vi "Pruebas-VER1.1.vi"() -> ()   [LabVIEW 2020]
uses:
  <vilib>/Instr/_visa.llb/VISA Open Access Mode.ctl
  <vilib>/Instr/_visa.llb/VISA Configure Serial Port (Instr).vi
panel:
  out "Numeric":i32
  in  "stop 2":bool
  in  "stop":bool
  out "Contador ciclos":i32
  in  "format string 3":string
  out "error out 2":errorcluster
  in  "Tab":enum32{"Datos Generales", "Calibración", "LVDT"}(tab) caption="Tab Control"
  in  "Número de muestra":string
  in  "Tab Control":enum32{"Contenido de Humedad ", " Anillo"}(tab)
  in  "Peso Tara (mr) [g]":string
  in  "Peso Suelo Seco + Tara (hora 1) (ms) [g]":string
  in  "Peso Suelo Seco + Tara (hora 0) (ms) [g]":string
  in  "Peso Suelo Húmedo + Tara (mh) [g]":string
  in  "Balanza N°":string
  in  "Cápsula N°":string
  in  "Balanza N°":string
  in  "Anillo N° [ANC-]":string
  in  "P. Anillo + muestra seca [g]":string
  in  "P. Anillo + Muestra sumergida [g]":string
  in  "P. Anillo + Muestra natural [g]":string
  in  "N° de brazo":string(combo)
  in  "Tipo de ensayo":string(combo)
  in  "Nombre del proyecto":string
  in  "Número de Ingreso":string
  in  "Operaria/o":string
  in  "Lugar donde se almacenará nuestro archivo":path
  in  "Save Button":bool
  in  "EST_CAL":string
  in  "Settings Button":bool
  in  "Nueva Configuración":dbl
  in  "Configuración":bool
  out "Hexadecimal":string
  out "Calibración Actual":dbl
  out "Defo (mm)":dbl
  out "microvolts":u32
  out "Voltaje (V)":dbl
  in  "Ingrese el valor de la carga":string
  in  "Obs Muestra":bool
  out "XY Graph":cluster{"X":dbl, "Y":dbl}[](graph)
  out "Actualización de tabla en tiempo real con deformación":string[][](table)
  in  "Observación de la muestra":string
  in  "Play Button":bool
  out "ciclo inicio":i32
  out "Voltaje (V) 2":dbl format="%#_8f"
  out "Deformación (mm)":dbl format="%#_6f"
  out "error out":errorcluster
  out "Microvolts":i32
  in  "Pause Button":bool
  in  "Cancel Button":bool
  # "Parámetros para calibración"
  # "Recuerde: Las observaciones van al final del ensayo para no perjudicar los demas datos"
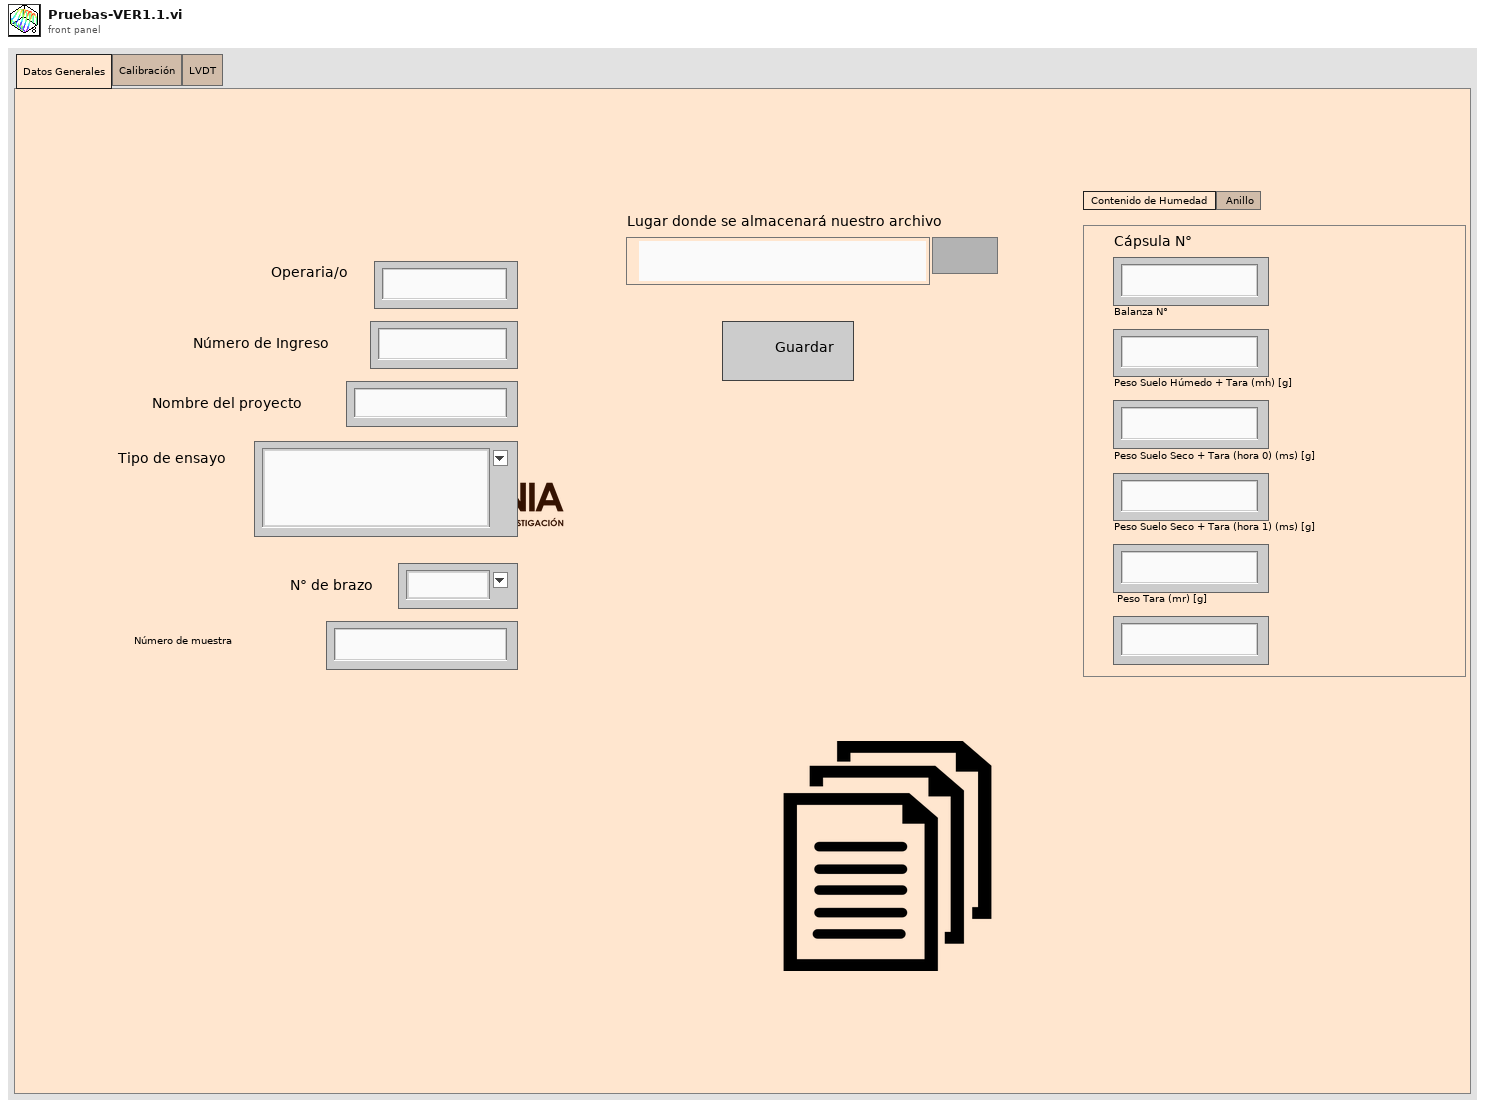
[diagram p1: front panel]
types:
  T1 = enum16{"open", "replace", "create", "open or create", "replace or create", "replace or create with confirmation"}
  T2 = typedef "VISA Open Access Mode.ctl" = u32
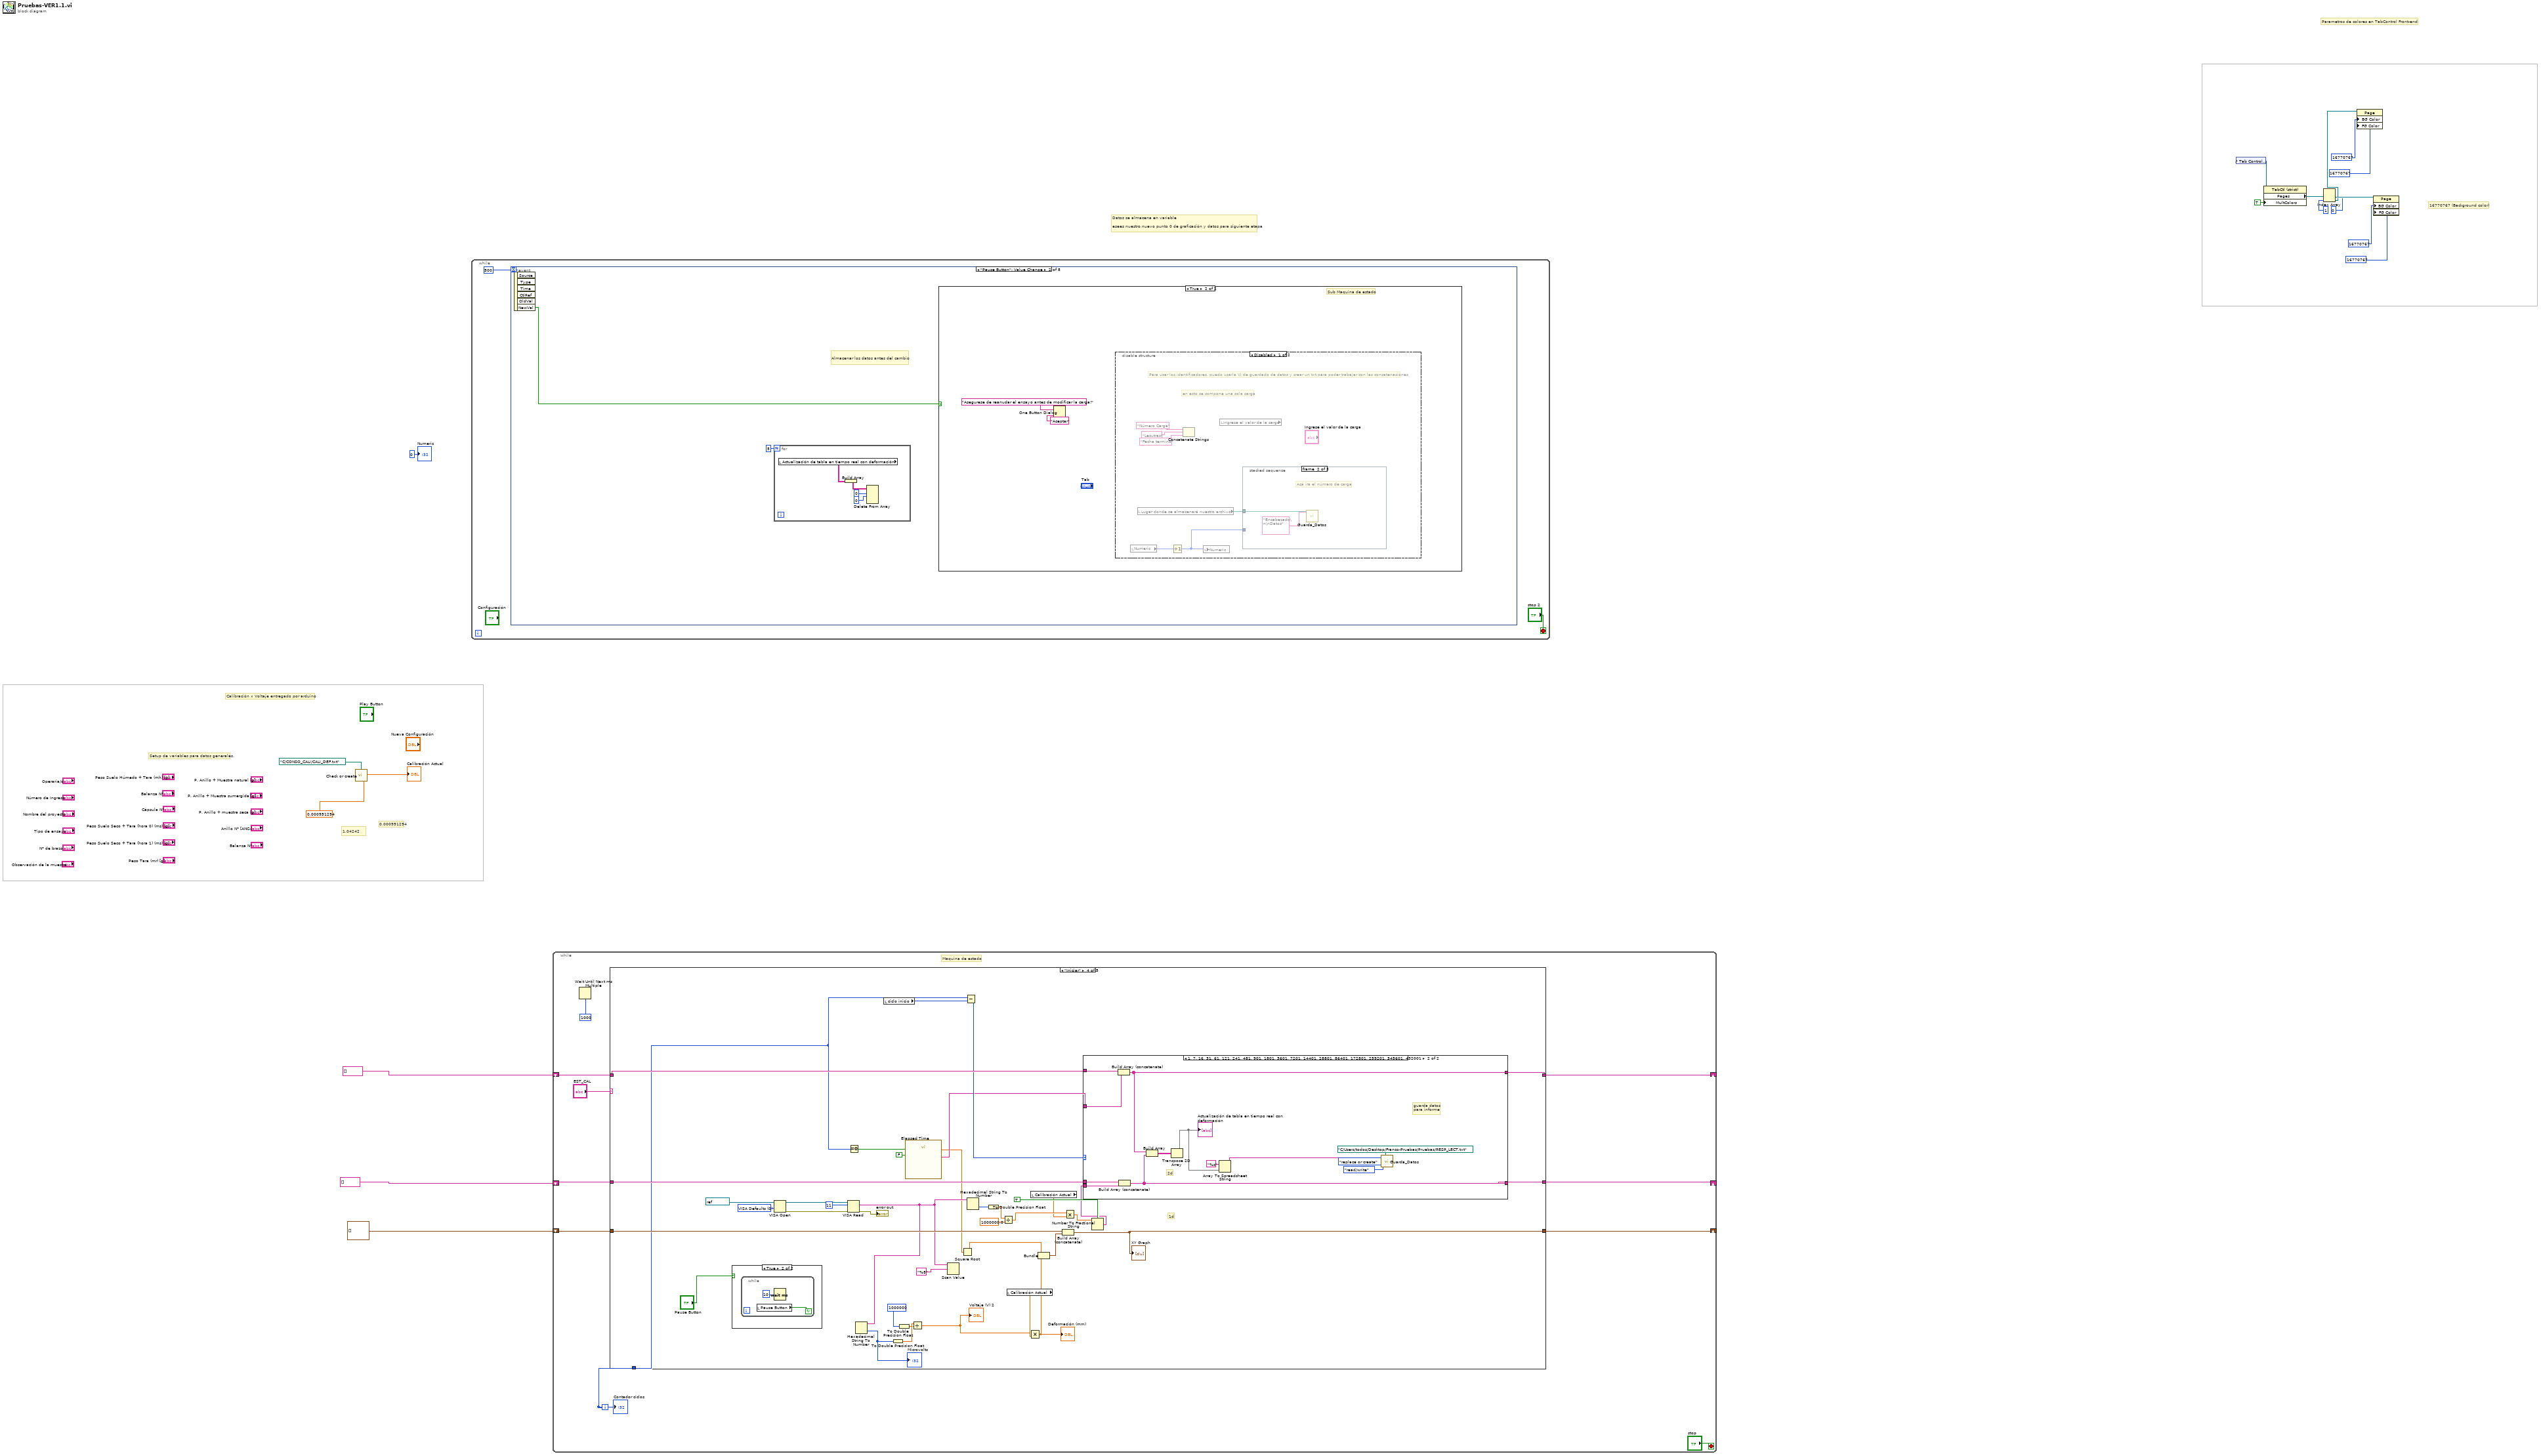
[diagram p0: block diagram]
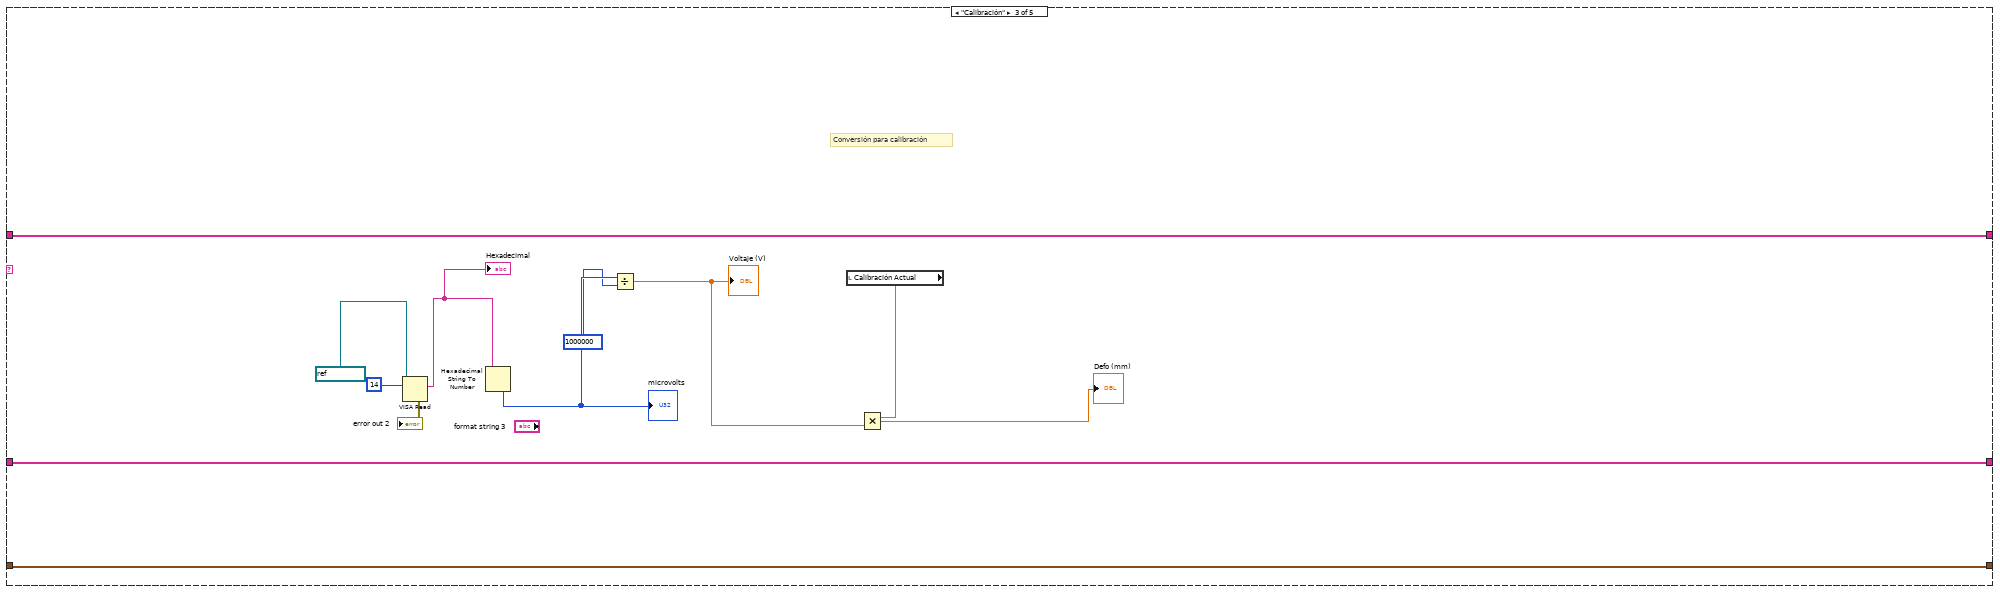
[diagram p4: hidden frame]
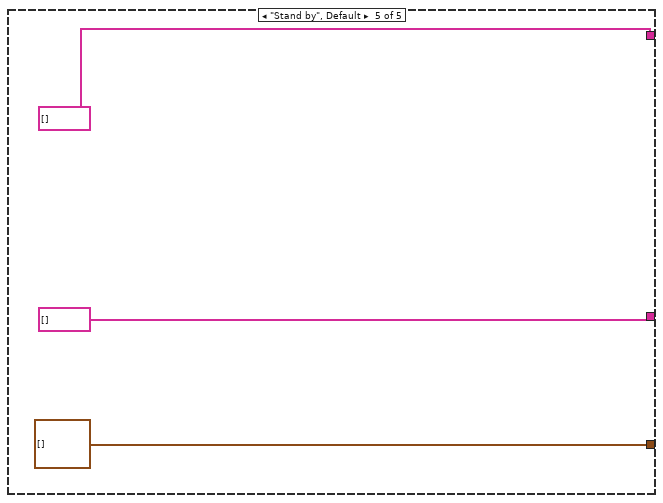
[diagram p7: hidden frame]
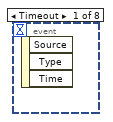
[diagram p8: hidden frame]
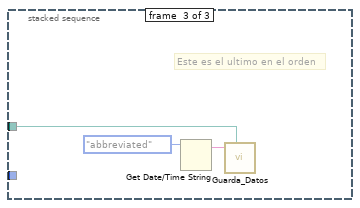
[diagram p11: hidden frame]
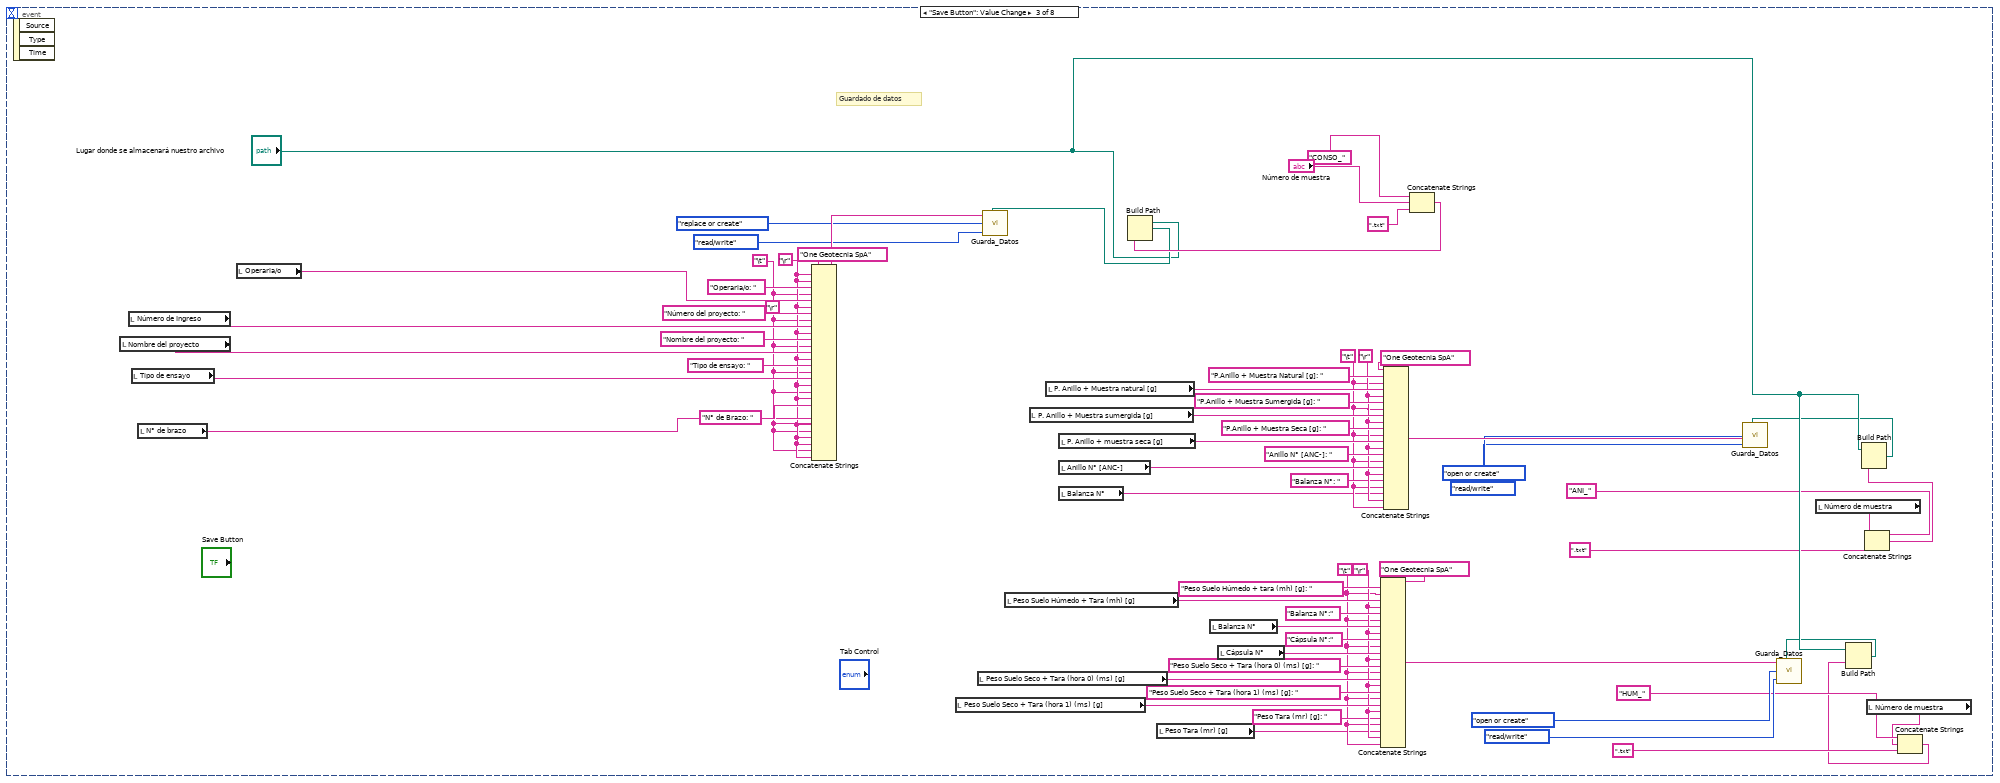
[diagram p13: hidden frame]
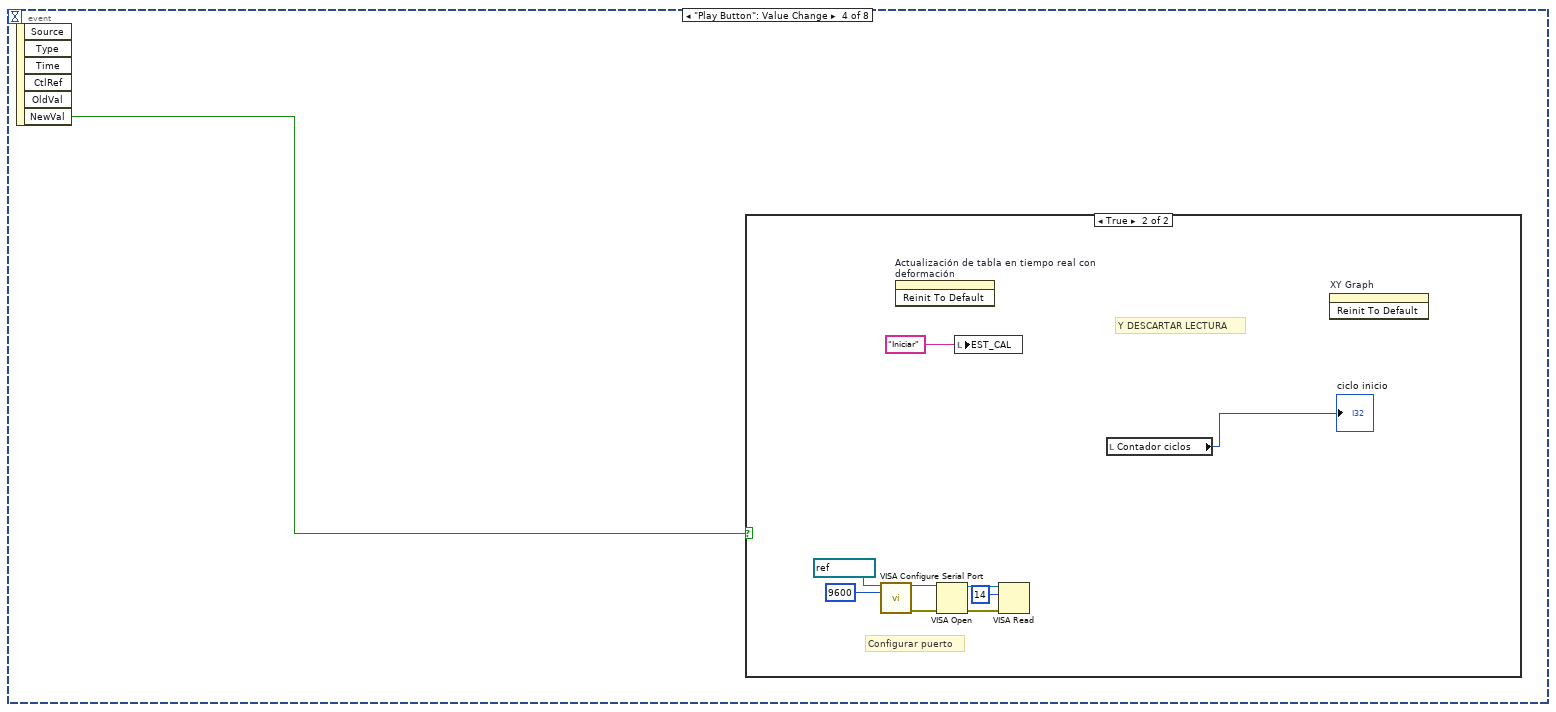
[diagram p14: hidden frame]
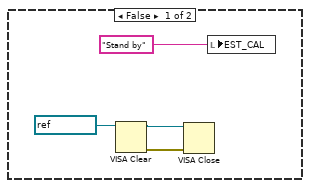
[diagram p15: hidden frame]
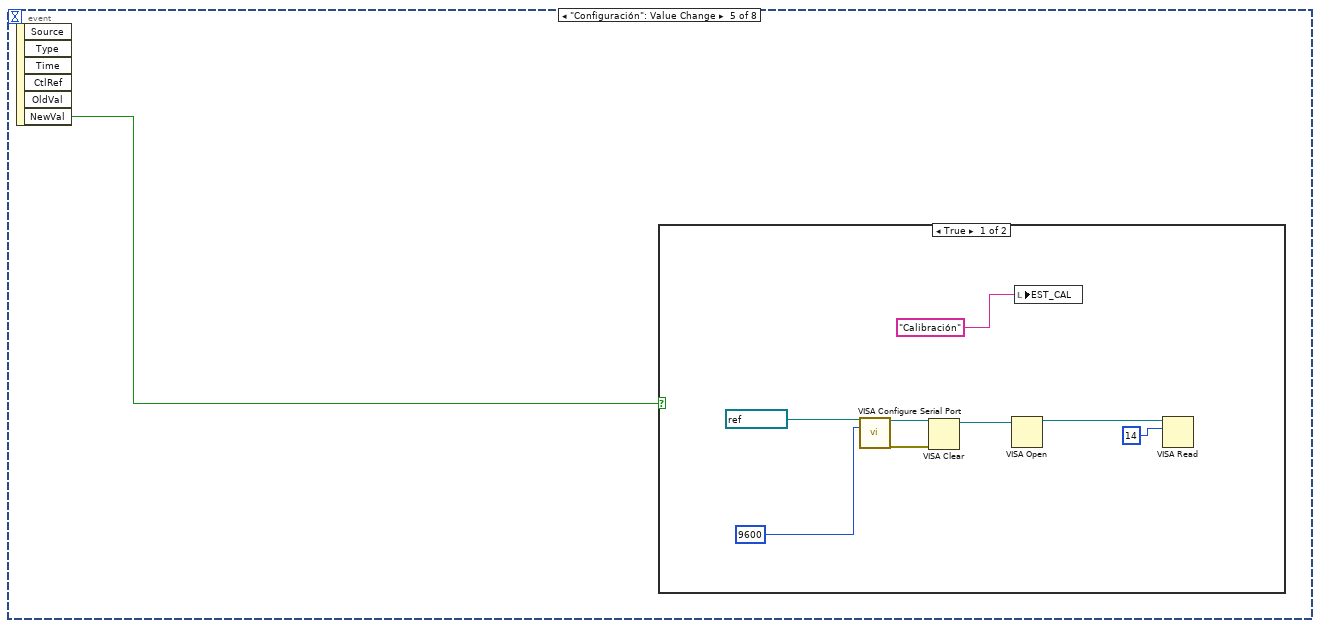
[diagram p16: hidden frame]
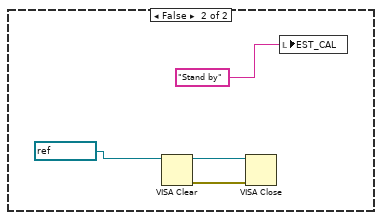
[diagram p17: hidden frame]
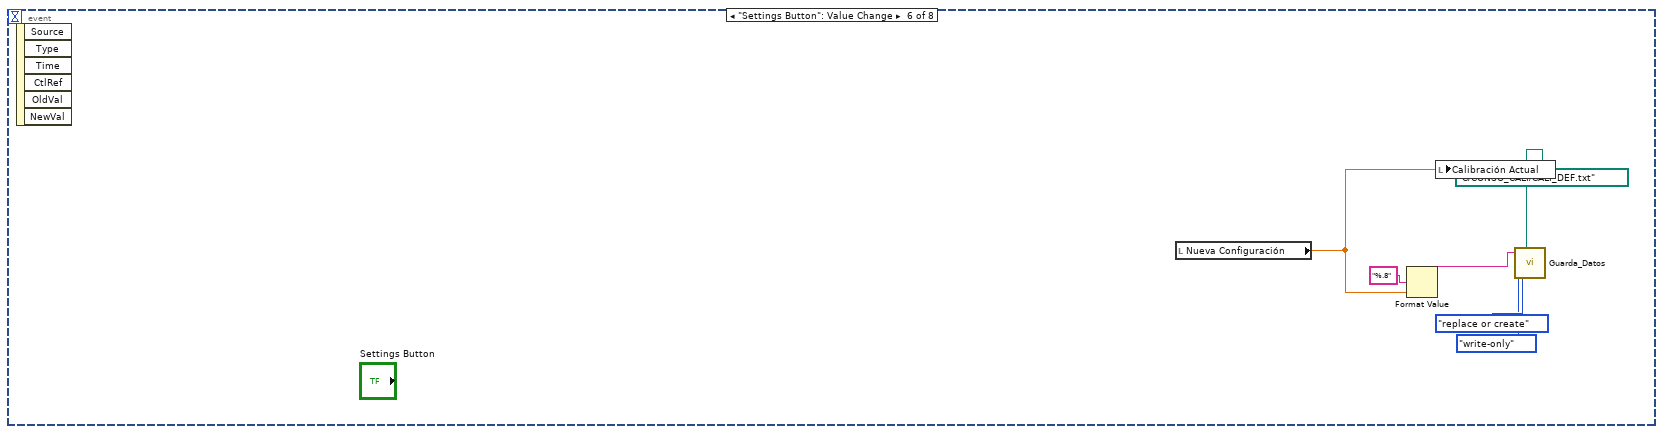
[diagram p18: hidden frame]
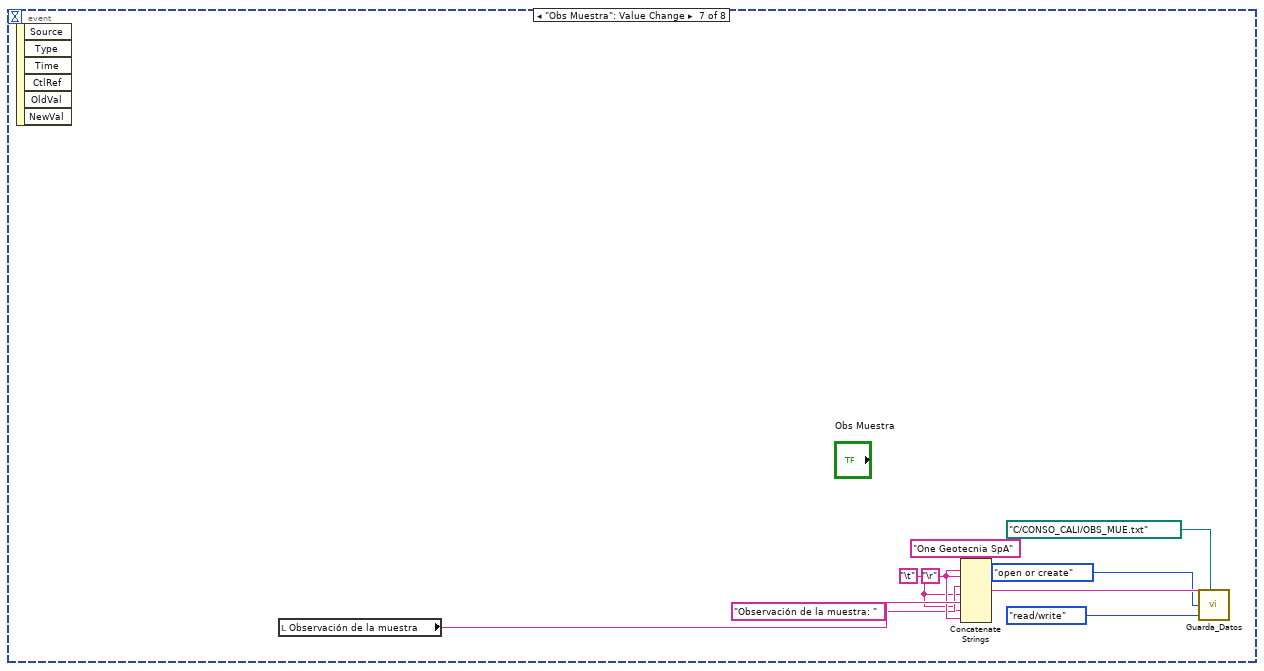
[diagram p19: hidden frame]
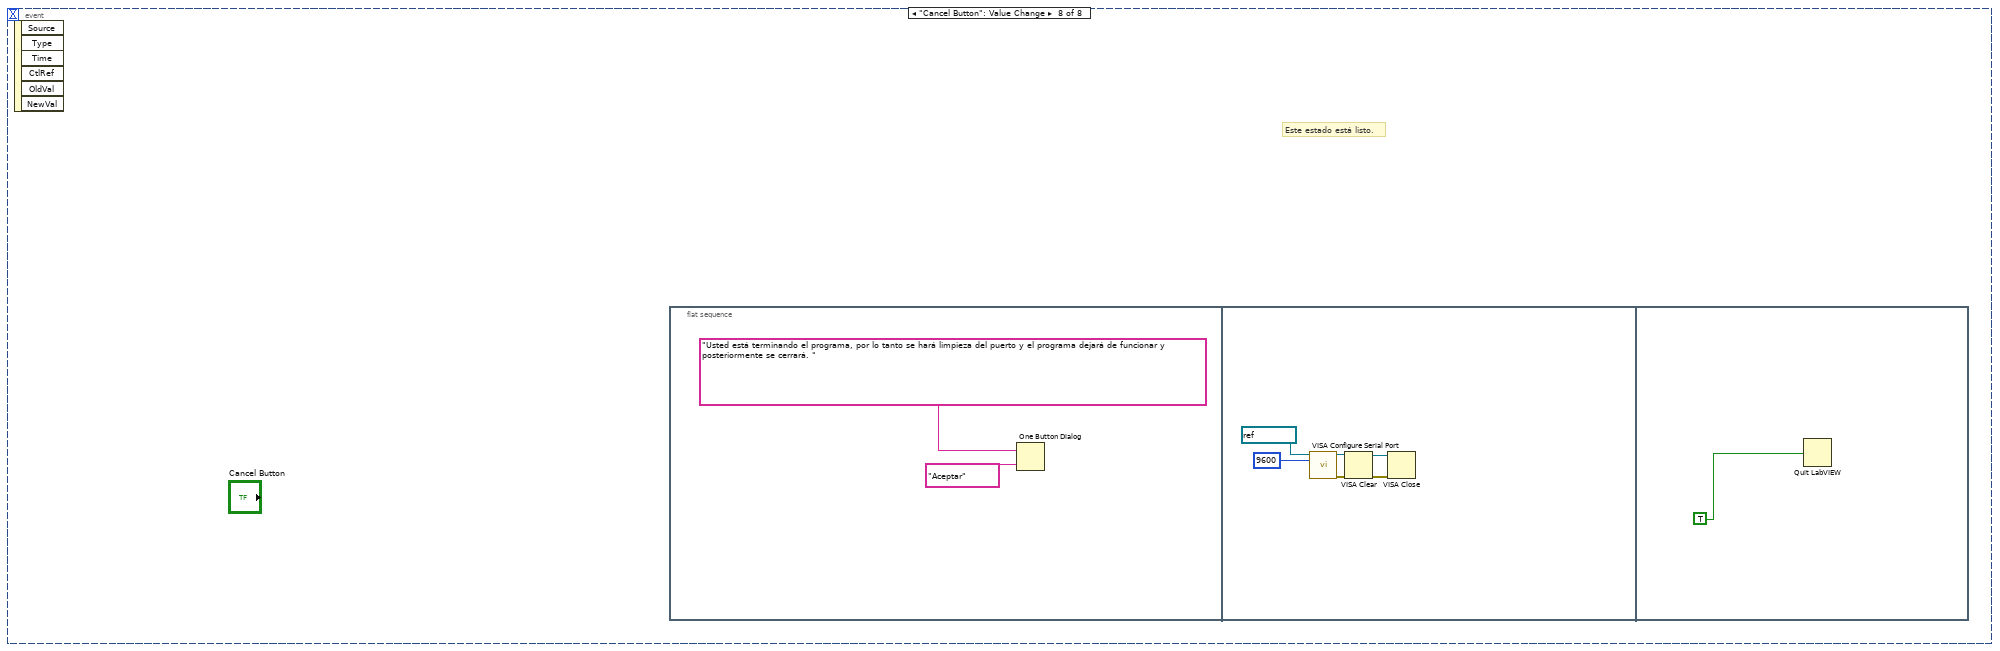
[diagram p20: hidden frame]
diagram:
  # "Datos se almacena en variable\n\nesees nuestro nuevo punto 0 de graficación y datos para siguiente etapa"
  # "1,04242"
  # "Calibración x Voltaje entregado por arduino"
  # "0,000951294"
  # "Setup de variables para datos generales."
  # "Parametros de colores en TabControl Front-end"
  # "16770767 (Background color)"
  n1 = call "Check or create.vi"("Default"=0.000951294, "Ruta"=path "C:/CONSO_CALI/CALI_DEF.txt") -> ("Valor guardado"=→"Calibración Actual":dbl)  [unwired: 8 in, 1 out]
  n2 = while {
    stop <- "stop 2" stop-if-true
    n3 = event shown="[1] \"Pause Button\": Value Change" {
      selector: _ -> [_ _ _ _ _ _ _ _]
      dyn-events: _ -> [_ _ _ _ _ _ _ _]
      timeout: 500 -> [_ _ _ _ _ _ _ _]
      event Timeout {
        n4 = event-data() -> ()  [unwired: 1 in, 3 out]
      }
      event "Pause Button": Value Change {
        # "Almacenar los datos antes del cambio"
        n5 = event-data() -> ("NewVal"=w22:bool)  [unwired: 1 in, 5 out]
        n6 = for {
          N: 5 -> [_]
          n7 = local read "Actualización de tabla en tiempo real con deformación"() -> (w25:string[][])
          n8 = Build Array(w25) -> (w26:string[][][])
          n9 = Delete From Array(array=w26, length=0, index (dim 0)=0 ("index (page)")) -> ()  [unwired: 2 in, 2 out]
        }
        n10 = case shown="True" w22 {
          frame False {
            # "Reseteo timer"
            # "Reseteo tabla"
          }
          frame True {
            # "Sub Maquina de estado"
            n11 = One Button Dialog(message="Asegurese de reanudar el ensayo antes de modificar la carga!", button name ("OK")="Aceptar") -> ()  [unwired: 1 out]
            n12 = disable-structure shown="Disabled" {
              frame Disabled {
                # "Para usar los identificadores, puedo usarla Vi de guardado de datos y crear un txt para poder trabajar con las concatenaciones"
                # "en esto se compone una sola carga"
                n13 = local read "Numeric"() -> (w34:i32)
                n14 = local read "Lugar donde se almacenará nuestro archivo"() -> (w29:path)
                n15 = Increment(x=w34) -> (x+1=w33:i32)
                n16 = Concatenate Strings("Número Carga" ("string"), "Lecutras" ("string"), "Fecha termino" ("string")) -> ()  [unwired: 1 out]
                n17 = local write "Numeric"(w33) -> ()
                n18 = local read "Ingrese el valor de la carga"() -> ()  [unwired: 1 out]
                n19 = stacked-sequence {
                  tunnel: w33 -> [_ _ _]
                  tunnel: w29 -> [_ w35 w37]
                  frame #0 {
                    # "Generar encabezado"
                    # "Generar ruta"
                  }
                  frame #1 {
                    # "Acá ira el número de carga"
                    n20 = call "Guarda_Datos.vi"("Texto (I)"="Encabezado\n\nDatos", "Ruta"=w35) -> ()  [unwired: 3 in, 2 out]
                  }
                  frame #2 {
                    # "Este es el ultimo en el orden"
                    n21 = Get Date/Time String(date format (0)=enum16{"short", "long", "abbreviated"}."abbreviated") -> (date string=w39:string)  [unwired: 2 in, 1 out]
                    n22 = call "Guarda_Datos.vi"("Texto (I)"=w39, "Ruta"=w37) -> ()  [unwired: 3 in, 2 out]
                  }
                }
              }
              frame Enabled {
              }
            }
          }
        }
      }
      event "Save Button": Value Change {
        (unwired) "\r"
        w65 = "\r"
        w63 = "\t"
        w83 = "\r"
        w81 = "\t"
        w94 = "\r"
        w93 = "\t"
        # "Guardado de datos"
        n23 = event-data() -> ()  [unwired: 1 in, 3 out]
        n24 = local read "Nombre del proyecto"() -> (w99:string)
        n25 = local read "Número de Ingreso"() -> (w101:string)
        n26 = local read "Tipo de ensayo"() -> (w97:string)
        n27 = local read "N° de brazo"() -> (w95:string)
        n28 = local read "Operaria/o"() -> (w103:string)
        n29 = Concatenate Strings("One Geotecnia SpA" ("element"), w94, w94, "Operaria/o: " ("element"), w93, w103, w94, "Número del proyecto: " ("element"), w93, w101, w94, "Nombre del proyecto: " ("element"), w93, w99, w94, "Tipo de ensayo: " ("element"), w93, w97, w94, w93, w94, "N° de Brazo: " ("element"), w93, w95, w94, w93, w94, w94, w93, w94) -> (w58:string)
        n30 = local read "Peso Suelo Seco + Tara (hora 1) (ms) [g]"() -> (w66:string)
        n31 = local read "Peso Suelo Seco + Tara (hora 0) (ms) [g]"() -> (w68:string)
        n32 = local read "Peso Suelo Húmedo + Tara (mh) [g]"() -> (w74:string)
        n33 = local read "P. Anillo + Muestra sumergida [g]"() -> (w88:string)
        n34 = local read "P. Anillo + Muestra natural [g]"() -> (w90:string)
        n35 = local read "P. Anillo + muestra seca [g]"() -> (w86:string)
        n36 = local read "Anillo N° [ANC-]"() -> (w84:string)
        n37 = local read "Balanza N°"() -> (w80:string)
        n38 = local read "Peso Tara (mr) [g]"() -> (w62:string)
        n39 = local read "Balanza N°"() -> (w72:string)
        n40 = local read "Cápsula N°"() -> (w70:string)
        n41 = Concatenate Strings("One Geotecnia SpA" ("element"), "Peso Suelo Húmedo + tara (mh) [g]: " ("string"), w63, w74, w65, "Balanza N°:" ("string"), w63, w72, w65, "Cápsula N°:" ("string"), w63, w70, w65, "Peso Suelo Seco + Tara (hora 0) (ms) [g]: " ("string"), w63, w68, w65, "Peso Suelo Seco + Tara (hora 1) (ms) [g]: " ("string"), w63, w66, w65, "Peso Tara (mr) [g]: " ("string"), w63, w62, w65, w63) -> (w61:string)
        n42 = Concatenate Strings("One Geotecnia SpA" ("element"), "P.Anillo + Muestra Natural [g]: " ("string"), w81, w90, w83, "P.Anillo + Muestra Sumergida [g]: " ("string"), w81, w88, w83, "P.Anillo + Muestra Seca [g]: " ("string"), w81, w86, w83, "Anillo N° [ANC-]: " ("string"), w81, w84, w83, "Balanza N°: " ("string"), w81, w80, w83, w81) -> (w79:string)
        n43 = Concatenate Strings("CONSO_", "Número de muestra", ".txt" ("string")) -> (w52:string)
        n44 = Build Path(base path="Lugar donde se almacenará nuestro archivo", name or relative path=w52) -> (appended path=w51:path)
        n45 = call "Guarda_Datos.vi"("Texto (I)"=w58, "Ruta"=w51, "Operación"=T1."replace or create", "Acceso"=enum16{"read/write", "read-only", "write-only"}."read/write") -> ()  [unwired: 1 in, 2 out]
        n46 = local read "Número de muestra"() -> (w48:string)
        n47 = Concatenate Strings("ANI_" ("string"), w48, ".txt" ("string")) -> (w44:string)
        n48 = Build Path(base path="Lugar donde se almacenará nuestro archivo", name or relative path=w44) -> (appended path=w40:path)
        n49 = call "Guarda_Datos.vi"("Texto (I)"=w79, "Ruta"=w40, "Operación"=T1."open or create", "Acceso"=enum16{"read/write", "read-only", "write-only"}."read/write") -> ()  [unwired: 1 in, 2 out]
        n50 = local read "Número de muestra"() -> (w47:string)
        n51 = Concatenate Strings("HUM_" ("string"), w47, ".txt" ("string")) -> (w42:string)
        n52 = Build Path(base path="Lugar donde se almacenará nuestro archivo", name or relative path=w42) -> (appended path=w41:path)
        n53 = call "Guarda_Datos.vi"("Texto (I)"=w61, "Ruta"=w41, "Operación"=T1."open or create", "Acceso"=enum16{"read/write", "read-only", "write-only"}."read/write") -> ()  [unwired: 1 in, 2 out]
      }
      event "Play Button": Value Change {
        n54 = event-data() -> ("NewVal"=w106:bool)  [unwired: 1 in, 5 out]
        n55 = case shown="True" w106 {
          frame False {
            n56 = VISA Clear(VISA resource name=refnum<visa-resource-name> "COM3") -> (VISA resource name out=w108:refnum<visa-resource-name>, error out=w107:errorcluster)  [unwired: 1 in]
            n57 = VISA Close(VISA resource name=w108, error in (no error)=w107) -> ()  [unwired: 1 out]
            n58 = local write "EST_CAL"("Stand by" ("INI_E")) -> ()
          }
          frame True {
            # "Y DESCARTAR LECTURA"
            # "Configurar puerto"
            n59 = call-poly "VISA Configure Serial Port"("VISA resource name"=refnum<visa-resource-name> "COM3", "baud rate (9600)"=u32 9600) -> ("VISA resource name out"=w115:refnum<visa-resource-name>, "error out"=w114:errorcluster)  [unwired: 12 in]
            n60 = invoke on="Actualización de tabla en tiempo real con deformación" class="Tbl (strict)" method="Reinit To Default"() -> ()  [unwired: 3 in, 3 out]
            n61 = VISA Open(error in (no error)=w114, VISA resource name=w115) -> (VISA resource name=w113:refnum<visa-resource-name>, error out=w112:errorcluster)  [unwired: 3 in]
            n62 = local write "EST_CAL"("Iniciar" ("INI_E")) -> ()
            n63 = VISA Read(VISA resource name=w113, byte count=u32 14, error in (no error)=w112) -> ()  [unwired: 4 out]
            n64 = local read "Contador ciclos"() -> (→"ciclo inicio":i32)
            n65 = invoke on="XY Graph" class="XYGraph (strict)" method="Reinit To Default"() -> ()  [unwired: 3 in, 3 out]
          }
        }
      }
      event "Configuración": Value Change {
        n66 = event-data() -> ("NewVal"=w120:bool)  [unwired: 1 in, 5 out]
        n67 = case shown="True" w120 {
          frame True {
            n68 = call-poly "VISA Configure Serial Port"("VISA resource name"=refnum<visa-resource-name> "COM3", "baud rate (9600)"=u32 9600) -> ("VISA resource name out"=w124:refnum<visa-resource-name>, "error out"=w121:errorcluster)  [unwired: 12 in]
            n69 = VISA Clear(VISA resource name=w124, error in (no error)=w121) -> (VISA resource name out=w123:refnum<visa-resource-name>)  [unwired: 1 out]
            n70 = VISA Open(VISA resource name=w123) -> (VISA resource name=w122:refnum<visa-resource-name>)  [unwired: 4 in, 1 out]
            n71 = local write "EST_CAL"("Calibración" ("EST_CAL")) -> ()
            n72 = VISA Read(VISA resource name=w122, byte count=u32 14) -> ()  [unwired: 1 in, 4 out]
          }
          frame False {
            n73 = VISA Clear(VISA resource name=refnum<visa-resource-name> "COM3") -> (VISA resource name out=w131:refnum<visa-resource-name>, error out=w130:errorcluster)  [unwired: 1 in]
            n74 = VISA Close(VISA resource name=w131, error in (no error)=w130) -> ()  [unwired: 1 out]
            n75 = local write "EST_CAL"("Stand by" ("EST_CAL")) -> ()
          }
        }
      }
      event "Settings Button": Value Change {
        n76 = event-data() -> ()  [unwired: 1 in, 6 out]
        n77 = local read "Nueva Configuración"() -> (w133:dbl)
        n78 = Format Value(format string="%.8", value (0)=w133) -> (output string=w135:string)  [unwired: 1 in]
        n79 = local write "Calibración Actual"(w133) -> ()
        n80 = call "Guarda_Datos.vi"("Texto (I)"=w135, "Ruta"=path "C:/CONSO_CALI/CALI_DEF.txt", "Operación"=T1."replace or create", "Acceso"=enum16{"read/write", "read-only", "write-only"}."write-only") -> ()  [unwired: 1 in, 2 out]
      }
      event "Obs Muestra": Value Change {
        w142 = "\r"
        w140 = "\t"
        n81 = event-data() -> ()  [unwired: 1 in, 6 out]
        n82 = local read "Observación de la muestra"() -> (w147:string)
        n83 = Concatenate Strings("One Geotecnia SpA" ("string"), w142, w142, "Observación de la muestra: " ("element"), w140, w147, w140, w142) -> (w146:string)
        n84 = call "Guarda_Datos.vi"("Texto (I)"=w146, "Ruta"=path "C:/CONSO_CALI/OBS_MUE.txt", "Operación"=T1."open or create", "Acceso"=enum16{"read/write", "read-only", "write-only"}."read/write") -> ()  [unwired: 1 in, 2 out]
      }
      event "Cancel Button": Value Change {
        # "Este estado está listo."
        n85 = event-data() -> ()  [unwired: 1 in, 6 out]
        n86 = flat-sequence {
          frame #0 {
            n87 = One Button Dialog(message="Usted está terminando el programa, por lo tanto se hará limpieza del puerto y el programa dejará de funcionar y posteriormente se cerrará. ", button name ("OK")="Aceptar") -> ()  [unwired: 1 out]
          }
          frame #1 {
            n88 = call-poly "VISA Configure Serial Port"("VISA resource name"=refnum<visa-resource-name> "COM3", "baud rate (9600)"=u32 9600) -> ("VISA resource name out"=w154:refnum<visa-resource-name>, "error out"=w155:errorcluster)  [unwired: 12 in]
            n89 = VISA Clear(VISA resource name=w154, error in (no error)=w155) -> (VISA resource name out=w153:refnum<visa-resource-name>, error out=w152:errorcluster)
            n90 = VISA Close(VISA resource name=w153, error in (no error)=w152) -> ()  [unwired: 1 out]
          }
          frame #2 {
            n91 = Quit LabVIEW(quit? (T)=TRUE ("Cancel Button")) -> ()
          }
        }
      }
    }
  }
  n92 = while {
    shift-right: [w164] -> _
    shift-left: cluster{dbl, dbl}[] [] -> [w165]
    shift-right: [w163] -> _
    shift-left: string[] [] ("appended array") -> [w162]
    shift-right: [w161] -> _
    shift-left: string[] [] ("appended array") -> [w160]
    i -> [w159]
    stop <- "stop" stop-if-true
    # "Maquina de estado"
    n93 = Wait Until Next ms Multiple(millisecond multiple=u32 1000) -> ()  [unwired: 1 out]
    n94 = case shown="\"Iniciar\"" "EST_CAL" {
      tunnel: w165 -> [w167 w170 w181 w223 _]
      tunnel: [w167 w170 w181 w222 cluster{dbl, dbl}[] []] -> w164
      tunnel: [w168 w171 w180 w221 string[] [] ("appended array")] -> w163
      tunnel: w162 -> [w168 w171 w180 w220 _]
      tunnel: [w169 w172 w179 w209 string[] [] ("appended array")] -> w161
      tunnel: w160 -> [w169 w172 w179 w219 _]
      tunnel: w159 -> [_ _ _ w210 _]
      frame "Pausa" {
      }
      frame "False" {
      }
      frame "Calibración" {
        # "Conversión para calibración"
        n95 = VISA Read(VISA resource name=refnum<visa-resource-name> "COM3", byte count=u32 14) -> (read buffer=w178:string, error out=→"error out 2":errorcluster)  [unwired: 1 in, 2 out]
        "Hexadecimal" <- w178
        n96 = Hexadecimal String To Number(string=w178) -> (number=w177:u32)  [unwired: 2 in, 1 out]
        "microvolts" <- w177
        n97 = Divide(x=w177, y=u32 1000000 ("x")) -> (x/y=w173:dbl)
        "Voltaje (V)" <- w173
        n98 = local read "Calibración Actual"() -> (w174:dbl)
        n99 = Multiply(x=w174, y=w173) -> (x*y=→"Defo (mm)":dbl)
      }
      frame "Iniciar" {
        w200 = T2 0 items=["VISA Defaults"=0, "Exclusive Lock"=1, "Load Configured Settings"=4] ("Access Mode")
        # "1d"
        n100 = case shown="True" "Pause Button" {
          frame False {
          }
          frame True {
            n101 = while {
              stop <- w225 continue-if-true
              n102 = local read "Pause Button"() -> (w225:bool)
              n103 = Wait (ms)(milliseconds to wait=u32 10) -> ()  [unwired: 1 out]
            }
          }
        }
        n104 = VISA Open(access mode=w200, VISA resource name=refnum<visa-resource-name> "COM3") -> (VISA resource name=w206:refnum<visa-resource-name>, error out=w199:errorcluster)  [unwired: 3 in]
        n105 = VISA Read(VISA resource name=w206, byte count=u32 11, error in (no error)=w199) -> (read buffer=w197:string, error out=→"error out":errorcluster)  [unwired: 2 out]
        n106 = Equal To 0?(x=w210) -> (x = 0?=w213:bool)
        n107 = Hexadecimal String To Number(string=w197) -> (number=w198:u32)  [unwired: 2 in, 1 out]
        "Microvolts" <- w198
        n108 = local read "ciclo inicio"() -> (w212:i32)
        n109 = To Double Precision Float(number=w198) -> (double precision float=w205:dbl)
        n110 = To Double Precision Float(number=1000000) -> (double precision float=w204:dbl)
        n111 = call "Elapsed Time"("Reset"=w213, "Auto Reset"=FALSE) -> ("Elapsed Time (s)"=w194:dbl, "Elapsed Time Text"=w195:string)  [unwired: 10 in, 6 out]
        n112 = Divide(x=w205, y=w204) -> (x/y=w201:dbl)
        "Voltaje (V) 2" <- w201
        n113 = Scan Value(string=w197, format string="%8") -> ()  [unwired: 1 in, 2 out]
        n114 = Square Root(x=w194) -> (sqrt(x)=w216:dbl)
        n115 = Subtract(x=w210, y=w212) -> (x-y=w211:i32)
        n116 = Hexadecimal String To Number(string=w197) -> (number=w192:u32)  [unwired: 2 in, 1 out]
        n117 = To Double Precision Float(number=w192) -> (double precision float=w189:dbl)
        n118 = Divide(x=w189, y=1000000.0) -> (x/y=w188:dbl)
        n119 = local read "Calibración Actual"() -> (w202:dbl)
        n120 = Multiply(x=w201, y=w202) -> (x*y=w196:dbl)
        "Deformación (mm)" <- w196
        n121 = local read "Calibración Actual"() -> (w187:dbl)
        n122 = Bundle(w216, w196) -> (w217:cluster{dbl, dbl})  [unwired: 1 in]
        n123 = Build Array (concatenate)(w223, w217) -> (w222:cluster{dbl, dbl}[])
        "XY Graph" <- w222
        n124 = Multiply(x=w188, y=w187) -> (x*y=w186:dbl)
        n125 = Number To Fractional String(use system decimal point (T)=TRUE, number=w186) -> (F-format string=w185:string)  [unwired: 2 in]
        n126 = case shown="1, 7, 16, 31, 61, 121, 241, 481, 901, 1801, 3601, 7201, 14401, 28801, 86401, 172801, 259201, 345601, 432001" w211 {
          tunnel: w220 -> [w226 w240]
          tunnel: w219 -> [w227 w239]
          tunnel: [w226 w238] -> w221
          tunnel: [w227 w237] -> w209
          tunnel: w195 -> [_ w236]
          tunnel: w185 -> [_ w234]
          frame 0, Default {
          }
          frame 1, 7, 16, 31, 61, 121, 241, 481, 901, 1801, 3601, 7201, 14401, 28801, 86401, 172801, 259201, 345601, 432001 {
            # "guarda datos\npara informe"
            # "2d"
            n127 = Build Array (concatenate)(w239, w236) -> (w237:string[])
            n128 = Build Array (concatenate)(w240, w234) -> (w238:string[])
            n129 = Build Array(w237, w238) -> (w235:string[][])
            n130 = Transpose 2D Array(2D array=w235) -> (transposed array=w228:string[][])
            "Actualización de tabla en tiempo real con deformación" <- w228
            n131 = Array To Spreadsheet String(array=w228, 3:"%s" ("format string")) -> (spreadsheet string=w233:string)  [unwired: 1 in]
            n132 = call "Guarda_Datos.vi"("Texto (I)"=w233, "Ruta"=path "C:/Users/todos/Desktop/Franco-Pruebas/Pruebas/RESP_LECT.txt", "Operación"=T1."replace or create", "Acceso"=enum16{"read/write", "read-only", "write-only"}."read/write") -> ()  [unwired: 1 in, 2 out]
          }
        }
      }
      frame "Stand by", Default {
      }
    }
    "Contador ciclos" <- w159
  }
  n133 = control-ref of="Tab Control Humedad"() -> (w16:refnum<vi>)
  n134 = property class="TabCtl (strict)"(reference=w16, "MultColors"=TRUE ("Allow Multiple Colors")) -> ("Pages"=w18:refnum<vi>[])  [unwired: 1 in, 2 out]
  n135 = Index Array(array=w18, index #1=0 ("index"), index #2=1 ("index")) -> (element #1=w17:refnum<vi>, element #2=w8:refnum<vi>)
  n136 = property class="Page"(reference=w8, "BG Color"=u32 16770767, "FG Color"=u32 16770767) -> ()  [unwired: 1 in, 2 out]
  n137 = property class="Page"(reference=w17, "BG Color"=u32 16770767, "FG Color"=u32 16770767) -> ()  [unwired: 1 in, 2 out]
  "Numeric" <- 0 ("Numeric")
